vi "Get Library File Path.vi"(10 "Class File Path":path) -> (2 "Library Path":path)   [LabVIEW 2021, in "_Shared.lvlib"]
uses:
  _Shared.lvlib
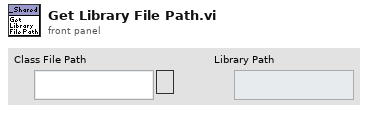
[diagram p1: front panel]
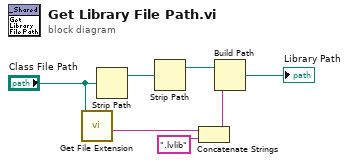
[diagram p0: block diagram]
diagram:
  n1 = call <vilib>:"Get File Extension.vi"("file"="Class File Path") -> ("filename without extension"=w5:string)  [unwired: 6 in, 4 out]
  n2 = Strip Path(path="Class File Path") -> (stripped path=w7:path)  [unwired: 1 out]
  n3 = Strip Path(path=w7) -> (stripped path=w6:path)  [unwired: 1 out]
  n4 = Concatenate Strings(w5, ".lvlib" ("string")) -> (w4:string)
  n5 = Build Path(base path=w6, name or relative path=w4) -> (appended path=→"Library Path":path)
